vi "Log Data.vi"(8 "error in (no error)":errorcluster, 10 "Data Queue":refnum<queue>, 11 "Logging Configuration":T1) -> (0 "error out":errorcluster)   [LabVIEW 2022 SP3, in "Logging.lvlib"]
doc: "This VI uses the TDMS Write function to write data to a TDMS file."
uses:
  Logging.lvlib
  <vilib>/Waveform/WDTFileIO.llb/Export Waveforms To Spreadsheet File (1D).vi
  Logging Configuration.ctl
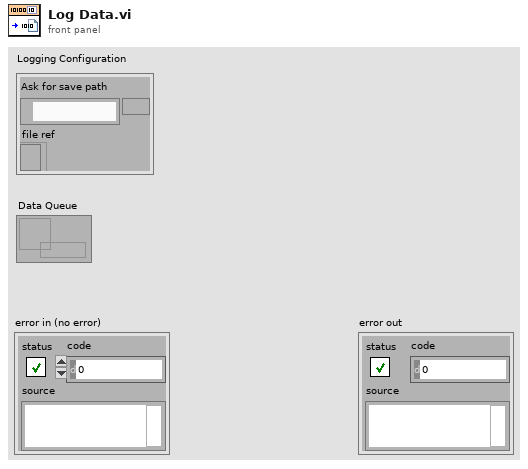
[diagram p1: front panel]
types:
  T1 = typedef "Logging.lvlib/Logging Configuration.ctl" = cluster{"Ask for save path":path, "file ref":refnum<file>}
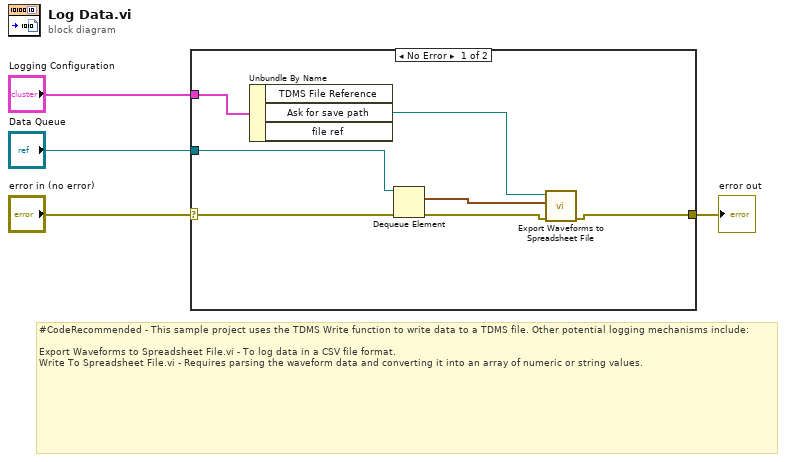
[diagram p0: block diagram]
diagram:
  # "#CodeRecommended - This sample project uses the TDMS Write function to write data to a TDMS file. Other potential logging mechanisms include:\n\nExport Waveforms to Spreadsheet File.vi - To log data in a CSV file format.\nWrite To Spreadsheet File.vi - Requires parsing the waveform data and converting it into an array of numeric or string values."
  n1 = case shown="No Error" "error in (no error)" {
    selector: "error in (no error)" -> [w10 w12]
    tunnel: "Logging Configuration" -> [w11 _]
    tunnel: "Data Queue" -> [w9 _]
    tunnel: [w5 w12] -> w2
    frame No Error {
      n2 = Unbundle By Name(w11) -> ("Ask for save path"=w7:path)  [unwired: 2 out]
      n3 = Dequeue Element(queue=w9, error in (no error)=w10) -> (element=w8:waveform(dbl)[], error out=w6:errorcluster)  [unwired: 1 in, 2 out]
      n4 = call-poly <vilib>:"Export Waveforms to Spreadsheet File.vi"("error in (no error)"=w6, "waveforms"=w8, "file path (dialog if empty)"=w7) -> ("error out"=w5:errorcluster)  [unwired: 7 in, 1 out]
    }
    frame Error {
    }
  }
  "error out" <- w2
